vi "ProbingTestSemiAuto.vi"() -> ()   [LabVIEW 2018]
uses:
  <vilib>/userdefined/High Color/IMAQdx.ctl
  <vilib>/Utility/file.llb/Read Delimited Spreadsheet (DBL).vi
  <vilib>/Utility/file.llb/Read Delimited Spreadsheet (I64).vi
  <vilib>/vision/driver/NI_Vision_Acquisition_Software.lvlib
  <vilib>/vision/NI_Vision_Development_Module.lvlib
panel:
  in  "Camera Offset Y":dbl=1.7
  in  "Camera Offset X":dbl=-98.89
  in  "Move To Separation?":bool
  in  "Move To Contact?":bool
  in  "Begin":bool
  out "Image Out":T1(plugin-control)
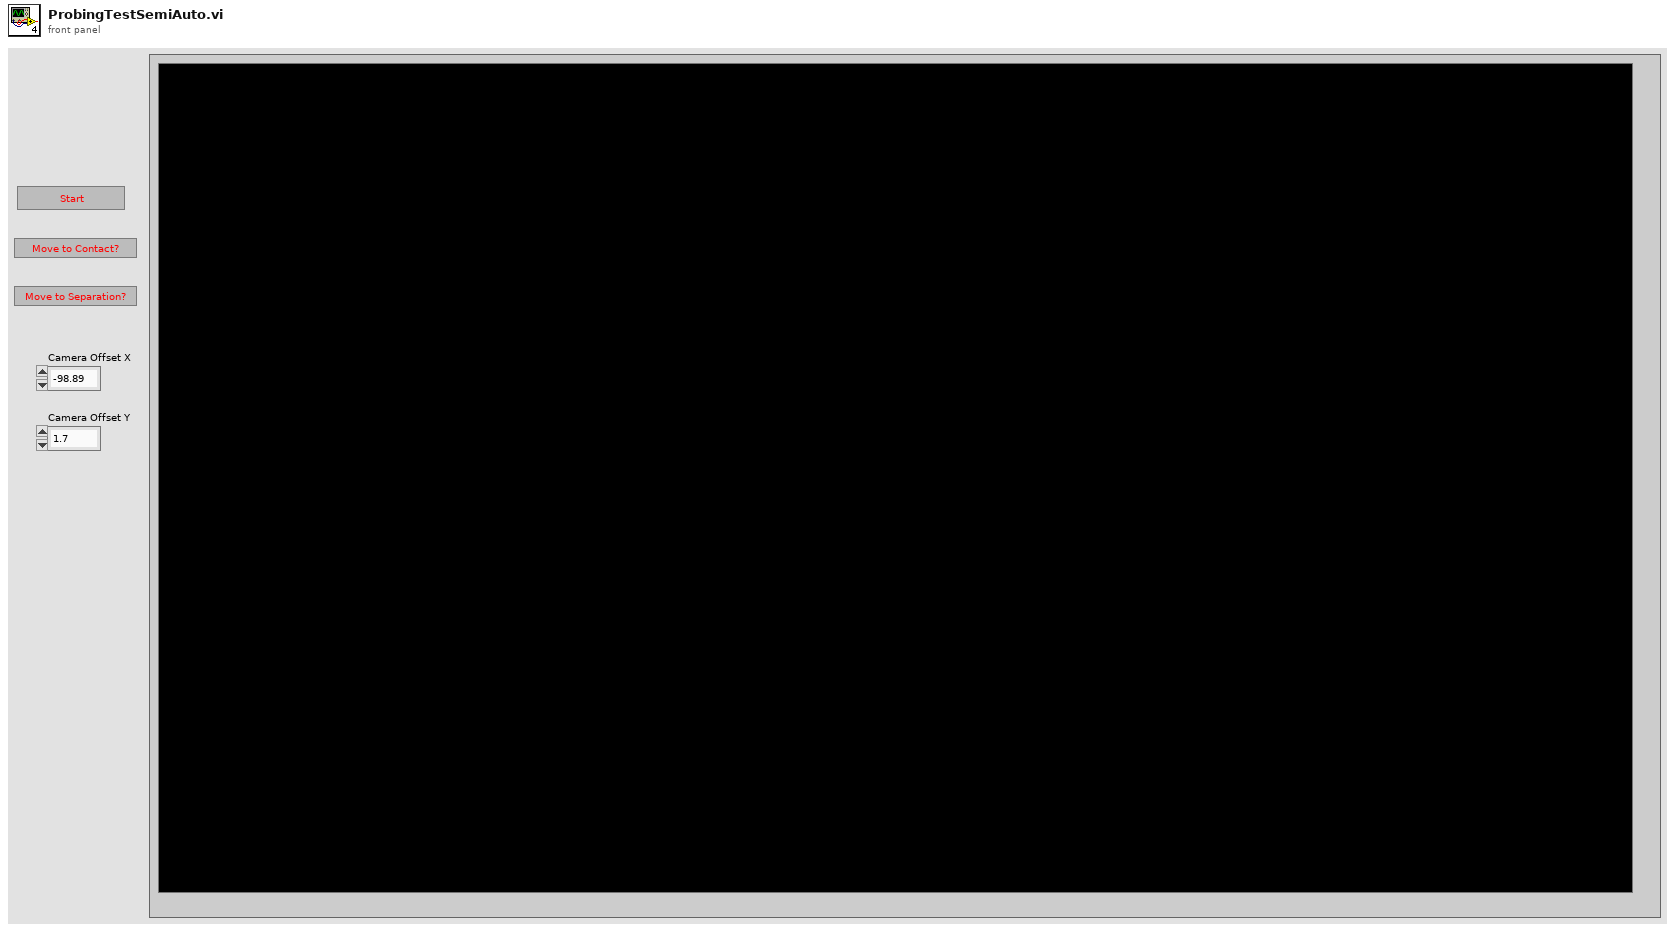
[diagram p1: front panel]
types:
  T1 = typedef "IMAQ Image.ctl" = refnum<image>
  T2 = typedef "Image Type" = u32
  T3 = typedef "IMAQdx.ctl" = refnum<k21>
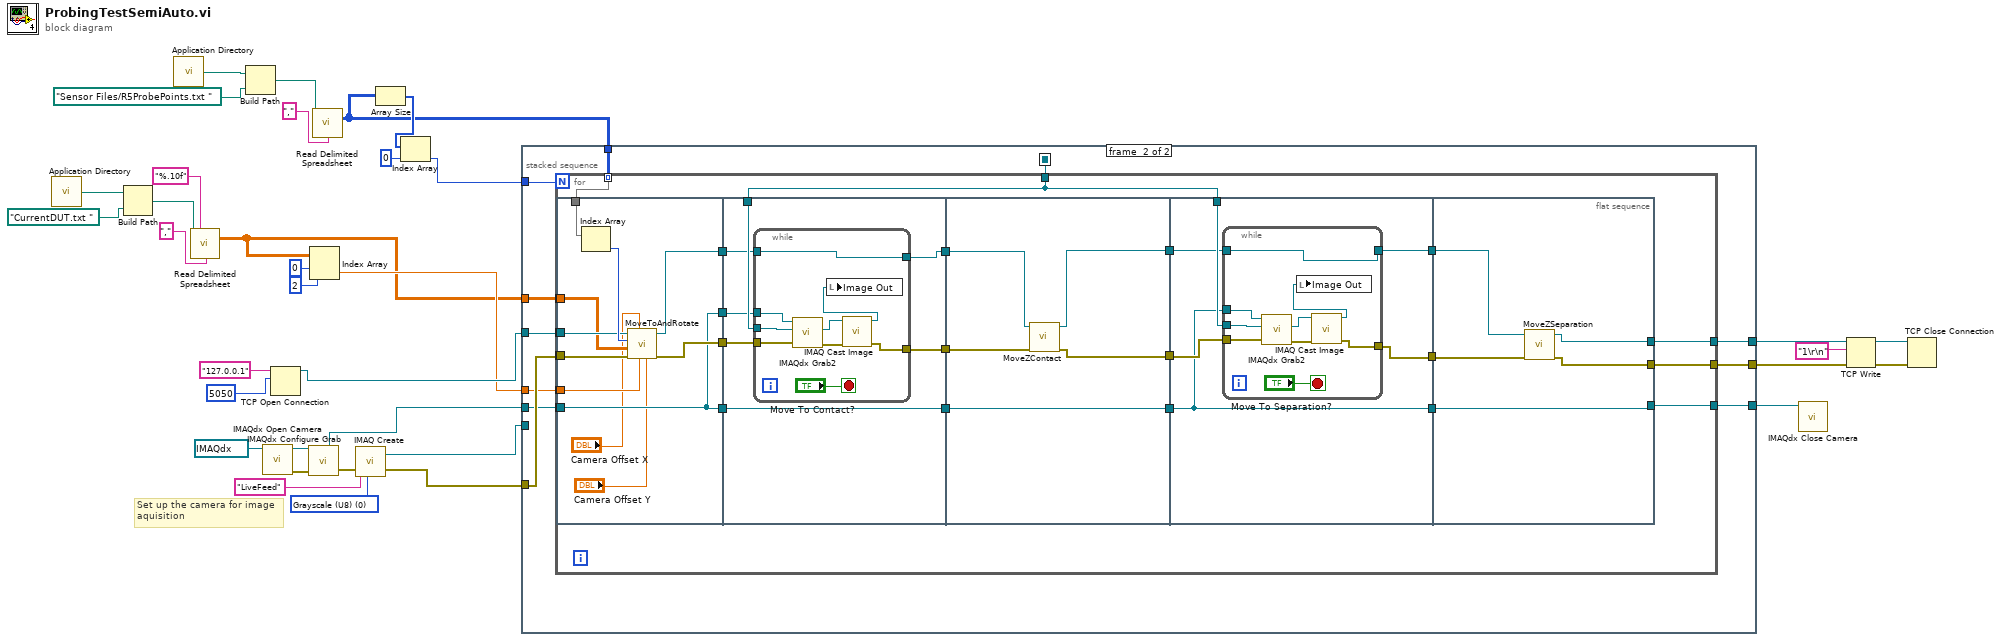
[diagram p0: block diagram]
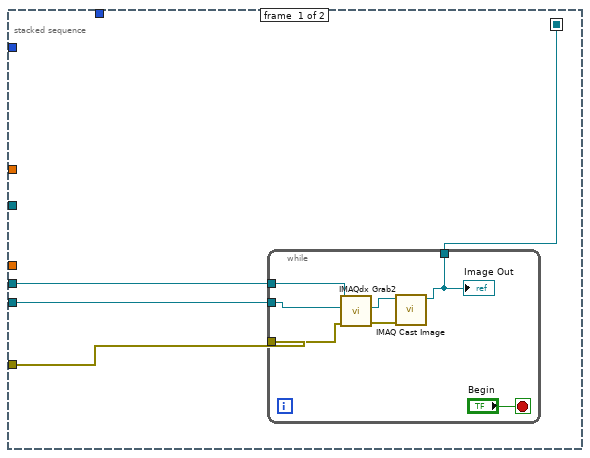
[diagram p2: hidden frame]
diagram:
  w25 = T2 0 items=["Grayscale (U8)", "Grayscale (I16)", "Grayscale (SGL)", "Complex (CSG)", "RGB (U32)", "HSL (U32)", "RGB (U64)", "Grayscale (U16)"] ("Image Type")
  # "Set up the camera for image \naquisition"
  n1 = call <vilib>:"Application Directory.vi"() -> ("Application Directory"=w32:path)
  n2 = Build Path(base path=w32, name or relative path=path "CurrentDUT.txt " ("file path (dialog if empty)")) -> (appended path=w33:path)
  n3 = call <vilib>:"Application Directory.vi"() -> ("Application Directory"=w1:path)
  n4 = call-poly <vilib>:"Read Delimited Spreadsheet.vi"("file path (dialog if empty)"=w33, "format (%.3f)"="%.10f", "delimiter (\\t)"="," ("delimiter (\\t)")) -> ("all rows"=w8:dbl[][])  [unwired: 7 in, 5 out]
  n5 = Build Path(base path=w1, name or relative path=path "Sensor Files/R5ProbePoints.txt " ("file path (dialog if empty)")) -> (appended path=w20:path)
  n6 = call <vilib>:"IMAQdx Open Camera.vi"("Session In"=T3 "cam0") -> ("error out"=w28:errorcluster, "Session Out"=w29:T3)  [unwired: 9 in]
  n7 = TCP Open Connection(address="127.0.0.1", remote port or service name=u16 5050) -> (connection ID=w10:refnum<k5>)  [unwired: 3 in, 1 out]
  n8 = call <vilib>:"IMAQdx Configure Grab.vi"("error in"=w28, "Session In"=w29) -> ("error out"=w26:errorcluster, "Session Out"=w15:T3)  [unwired: 8 in]
  n9 = Index Array(array=w8, index (row)=0, index (col)=2 ("disabled index (col)")) -> (element=w9:dbl)
  n10 = call-poly <vilib>:"Read Delimited Spreadsheet.vi"("file path (dialog if empty)"=w20, "delimiter (\\t)"="," ("delimiter (\\t)")) -> ("all rows"=w11:i64[][])  [unwired: 8 in, 5 out]
  n11 = call "IMAQ Create"("Image Name"="LiveFeed", "Image Type"=w25, "error in (no error)"=w26) -> ("New Image"=w14:T1, "error out"=w13:errorcluster)  [unwired: 2 in]
  n12 = Array Size(array=w11) -> (size(s)=w19:i32[])
  n13 = Index Array(array=w19, index=0) -> (element=w12:i32)
  n14 = stacked-sequence {
    seq-local: [w36 _] -> [_ w51]
    tunnel: w15 -> [w39 w50]
    tunnel: w14 -> [w38 _]
    tunnel: w13 -> [w37 w54]
    tunnel: w12 -> [_ w57]
    tunnel: w11 -> [_ w56]
    tunnel: w10 -> [_ w55]
    tunnel: w9 -> [_ w53]
    tunnel: w8 -> [_ w52]
    tunnel: [_ w49] -> w4
    tunnel: [_ w48] -> w3
    tunnel: [_ w47] -> w2
    frame #0 {
      n15 = while {
        tunnel: w39 -> [w45]
        tunnel: w38 -> [w41]
        tunnel: w37 -> [w40]
        tunnel: [w42] -> w36
        stop <- "Begin" stop-if-true
        n16 = call <vilib>:"IMAQdx Grab2.vi"("error in"=w40, "Image In"=w41, "Session In"=w45) -> ("error out"=w43:errorcluster, "Image Out"=w44:T1)  [unwired: 5 in, 2 out]
        n17 = call "IMAQ Cast Image"("error in (no error)"=w43, "Image Src"=w44) -> ("Image Dst Out"=w42:T1)  [unwired: 8 in, 1 out]
        "Image Out" <- w42
      }
    }
    frame #1 {
      n18 = for {
        N: w57 -> [_]
        tunnel: w51 -> [w69]
        tunnel: w56 -> [w80] mode=indexing
        tunnel: w55 -> [w79]
        tunnel: w54 -> [w78]
        tunnel: w53 -> [w77]
        tunnel: w52 -> [w76]
        tunnel: w50 -> [w74]
        tunnel: [w61] -> w49
        tunnel: [w60] -> w48
        tunnel: [w59] -> w47
        n19 = flat-sequence {
          tunnel: w80 -> [w91]
          tunnel: w79 -> [w89]
          tunnel: w78 -> [w88]
          tunnel: w77 -> [w87]
          tunnel: w76 -> [w86]
          tunnel: [w83] -> w75
          tunnel: w74 -> [w83]
          tunnel: [w85] -> w73
          tunnel: [w84] -> w72
          tunnel: [w83] -> w66
          tunnel: w69 -> [w98]
          tunnel: w75 -> [w97]
          tunnel: w73 -> [w96]
          tunnel: w72 -> [w92]
          tunnel: [w93] -> w71
          tunnel: [w95] -> w70
          tunnel: [w94] -> w67
          tunnel: w66 -> [w94]
          tunnel: w71 -> [w112]
          tunnel: w70 -> [w111]
          tunnel: [w110] -> w68
          tunnel: w67 -> [w110]
          tunnel: [w109] -> w65
          tunnel: [w108] -> w63
          tunnel: w69 -> [w118]
          tunnel: w68 -> [w115]
          tunnel: w65 -> [w117]
          tunnel: [w113] -> w64
          tunnel: w63 -> [w114]
          tunnel: [w116] -> w62
          tunnel: [w115] -> w58
          tunnel: w64 -> [w132]
          tunnel: w62 -> [w131]
          tunnel: [w130] -> w61
          tunnel: [w129] -> w60
          tunnel: [w128] -> w59
          tunnel: w58 -> [w128]
          frame #0 {
            n20 = Index Array(array=w91) -> (element=w90:i64)  [unwired: 1 in]
            n21 = call "MoveToAndRotate.vi"("Camera Offset Y"="Camera Offset Y", "Initial Angle"=w87, "Camera Offset X"="Camera Offset X", "Error In"=w88, "Probing Array"=w86, "Probe Index"=w90, "connection ID"=w89) -> ("error out"=w85:errorcluster, "connection ID 2"=w84:refnum<k5>)  [unwired: 3 in]
          }
          frame #1 {
            n22 = while {
              tunnel: w97 -> [w106]
              tunnel: w98 -> [w105]
              tunnel: w96 -> [w104]
              tunnel: [w100] -> w95
              tunnel: [w99] -> w93
              tunnel: w92 -> [w99]
              stop <- "Move To Contact?" stop-if-true
              n23 = call <vilib>:"IMAQdx Grab2.vi"("error in"=w104, "Image In"=w105, "Session In"=w106) -> ("error out"=w103:errorcluster, "Image Out"=w102:T1)  [unwired: 5 in, 2 out]
              n24 = call "IMAQ Cast Image"("error in (no error)"=w103, "Image Src"=w102) -> ("error out"=w100:errorcluster, "Image Dst Out"=w101:T1)  [unwired: 8 in]
              n25 = local write "Image Out"(w101) -> ()
            }
          }
          frame #2 {
            n26 = call "MoveZContact.vi"("error in (no error) 2"=w111, "connection ID 2"=w112) -> ("error out"=w109:errorcluster, "connection ID"=w108:refnum<k5>)  [unwired: 8 in]
          }
          frame #3 {
            n27 = while {
              tunnel: w115 -> [w126]
              tunnel: w118 -> [w125]
              tunnel: w117 -> [w124]
              tunnel: [w120] -> w116
              tunnel: [w119] -> w113
              tunnel: w114 -> [w119]
              stop <- "Move To Separation?" stop-if-true
              n28 = call <vilib>:"IMAQdx Grab2.vi"("error in"=w124, "Image In"=w125, "Session In"=w126) -> ("error out"=w123:errorcluster, "Image Out"=w122:T1)  [unwired: 5 in, 2 out]
              n29 = call "IMAQ Cast Image"("error in (no error)"=w123, "Image Src"=w122) -> ("error out"=w120:errorcluster, "Image Dst Out"=w121:T1)  [unwired: 8 in]
              n30 = local write "Image Out"(w121) -> ()
            }
          }
          frame #4 {
            n31 = call "MoveZSeparation.vi"("error in (no error) 2"=w131, "connection ID 2"=w132) -> ("error out"=w129:errorcluster, "connection ID"=w130:refnum<k5>)  [unwired: 8 in]
          }
        }
      }
    }
  }
  n32 = call <vilib>:"IMAQdx Close Camera.vi"("Session In"=w2) -> ()  [unwired: 10 in, 1 out]
  n33 = TCP Write(connection ID=w4, data in="1\r\n", error in (no error)=w3) -> (connection ID out=w6:refnum<k5>, error out=w7:errorcluster)  [unwired: 1 in, 1 out]
  n34 = TCP Close Connection(connection ID=w6, error in (no error)=w7) -> ()  [unwired: 1 in, 2 out]
